vi "Radians per Second to RPM.vi"   [LabVIEW 2017, in "NI_Robotics Utilities.lvlib"]
doc: "Converts an angular velocity from radians per second to rpm."
uses:
  <vilib>/robotics/Utilities/NI_Robotics Utilities.lvlib
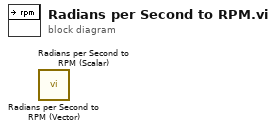
[diagram p0: block diagram]
diagram:
  n1 = call <vilib>:"Radians per Second to RPM (Vector).vi"() -> ()  [unwired: 3 in, 1 out]
  n2 = call <vilib>:"Radians per Second to RPM (Scalar).vi"() -> ()  [unwired: 3 in, 1 out]
